vi "Drive_sideways.vi"(4 "Buttons pushed?":bool) -> (1 "output":dbl format="%.2f", 2 "output angle":dbl)   [LabVIEW 2013]
uses:
  <vilib>/addons/control/pid/pid.llb/PID (DBL).vi
  <vilib>/addons/control/pid/NI_PID_pid.lvlib
panel:
  out "angle":dbl
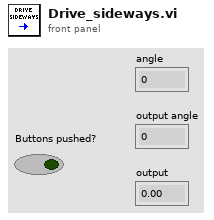
[diagram p1: front panel]
types:
  T1 = cluster{"proportional gain (Kc)":dbl, "integral time (Ti, min)":dbl, "derivative time (Td, min)":dbl}
  T2 = typedef "WPI_GyroDevRef.ctl" = cluster{"DevStatus":errorcluster, "Analog Module":T3, "Analog Channel":T4, "Offset":dbl, "Gain (VoltsPerDegree/Second)":dbl}
  T3 = typedef "FPGA_TypedefAnalogModule.ctl" = enum16{"Analog Module 1", "Analog Module 2"}
  T4 = typedef "FPGA_AIChannel.ctl" = enum8{"AI 1", "AI 2", "AI 3", "AI 4", "AI 5", "AI 6", "AI 7", "AI 8", "Invalid"}
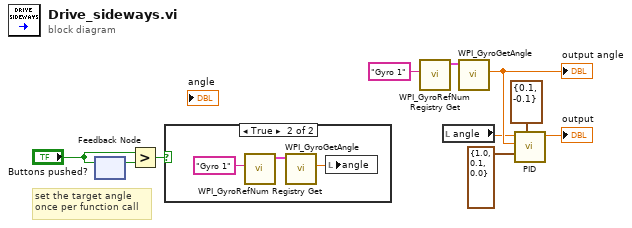
[diagram p0: block diagram]
diagram:
  # "set the target angle \nonce per function call"
  n1 = feedback #1() -> (w9:bool)  [unwired: 1 in]
  n2 = feedback-in #1("Buttons pushed?") -> ()
  n3 = Greater?(x="Buttons pushed?", y=w9) -> (0:w8:bool)
  n4 = case shown="True" w8 {
    frame False {
    }
    frame True {
      n5 = call <vilib>:"WPI_GyroRefNum Registry Get.vi"("refnum name"="Gyro 1") -> ("GyroDevRef"=w12:T2)  [unwired: 9 in, 1 out]
      n6 = call <vilib>:"WPI_GyroGetAngle.vi"("GyroDevRef"=w12) -> ("Angle"=w11:dbl)  [unwired: 7 in, 3 out]
      n7 = local write "angle"(w11) -> ()
    }
  }
  n8 = call <vilib>:"WPI_GyroRefNum Registry Get.vi"("refnum name"="Gyro 1") -> ("GyroDevRef"=w7:T2)  [unwired: 9 in, 1 out]
  n9 = local read "angle"() -> (w1:dbl)
  n10 = call <vilib>:"WPI_GyroGetAngle.vi"("GyroDevRef"=w7) -> ("Angle"=w2:dbl)  [unwired: 7 in, 3 out]
  "output angle" <- w2
  n11 = call-poly <vilib>:"PID.vi"("output range"=cluster{"output high":dbl, "output low":dbl} {"output high"=0.1, "output low"=-0.1}, "PID gains"=T1 {"proportional gain (Kc)"=1.0, "integral time (Ti, min)"=0.1, "derivative time (Td, min)"=0.0}, "process variable"=w2, "setpoint"=w1) -> ("output"=→"output":dbl)  [unwired: 6 in, 1 out]
